vi "Get Word Type.vi"(1 "Hash Function":refnum<class "NI_SHA-3.lvclass">) -> (0 "word type":T1 format="%016x")   [LabVIEW 2020, in "NI_SHA-3.lvclass"]
uses:
  <vilib>/security/Message Digest/SHA-3/NI_SHA-3.lvclass
  <vilib>/security/Message Digest/SHA-3/subVIs/state word.ctl
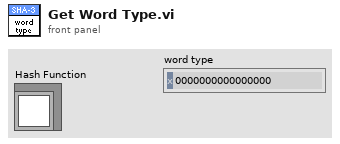
[diagram p1: front panel]
types:
  T1 = typedef "NI_SHA-3.lvclass/state word.ctl" = u64
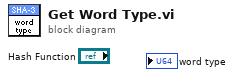
[diagram p0: block diagram]
diagram:
